vi "Did Command Change.vi"(9 "Paused":bool, 10 "Numeric":dbl, 11 "Ismatech 3 Channel Settings In":T1 {"Channel Number" min=0 max=3; "Pump Number" min=1}) -> (3 "Change":bool)   [LabVIEW 2018, in "Ismatec 4308.lvlib"]
uses:
  Ismatec 4308.lvlib
  Ismatec 4083.ctl
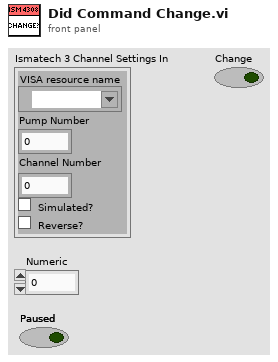
[diagram p1: front panel]
types:
  T1 = typedef "Ismatec 4308.lvlib/Ismatec 4083.ctl" = cluster{"VISA resource name":refnum<visa-resource-name>, "Pump Number":i16, "Channel Number":i16, "Simulated?":bool, "Reverse?":bool}
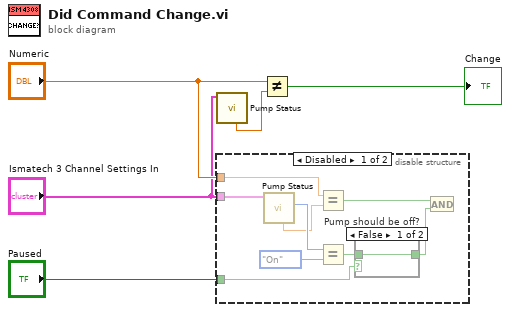
[diagram p0: block diagram]
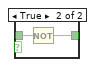
[diagram p2: hidden frame]
diagram:
  n1 = call "Pump Status.vi"("Ismatech 3 Channel Settings In"="Ismatech 3 Channel Settings In") -> ("RPM"=w3:dbl)  [unwired: 6 in, 4 out]
  n2 = disable-structure shown="Disabled" {
    disable-tunnel: "Paused" -> [w15 _]
    disable-tunnel: "Numeric" -> [w14 _]
    disable-tunnel: "Ismatech 3 Channel Settings In" -> [w8 _]
    frame Disabled {
      n3 = call "Pump Status.vi"("Ismatech 3 Channel Settings In"=w8) -> ("Pump On?"=w11:enum16{"Off", "On", "Not Initialized"}, "RPM"=w7:dbl)  [unwired: 6 in, 3 out]
      n4 = Equal?(x=w14, y=w7) -> (x = y?=w12:bool)
      n5 = Equal?(x=w11, y=enum16{"Off", "On", "Not Initialized"}."On") -> (x = y?=w10:bool)
      n6 = case "Pump should be off?" shown="False" w15 {
        tunnel: w10 -> [w16 w18]
        tunnel: [w16 w17] -> w13
        frame False {
        }
        frame True {
          n7 = Not(x=w18) -> (.not. x?=w17:bool)
        }
      }
      n8 = And(x=w12, y=w13) -> (x .and. y?=w6:bool)
    }
    frame Enabled {
    }
  }
  n9 = Not Equal?(x="Numeric", y=w3) -> (x != y?=→"Change":bool)
